vi "Create promotion move.vi"(9 "Destination":T1={"File"=enum."d", "Rank"=enum."4"}, 10 "Source":T1={"File"=enum."d", "Rank"=enum."4"}) -> (3 "Promotion move":refnum<class "Promotion.lvclass">)   [LabVIEW 2016, in "Chesslib.lvlib" / "Promotion.lvclass"]
uses:
  Promotion.lvclass
  C:/Users/GRTaggJ/Documents/Projects/chesslib/Moves/Move/Move.lvclass
  typedef/Square.ctl
  typedef/File.ctl
  typedef/Rank.ctl
  Promotion piece.ctl
  Promotion.lvclass/Promotion.ctl
  Move/Move.lvclass
  Chesslib.lvlib
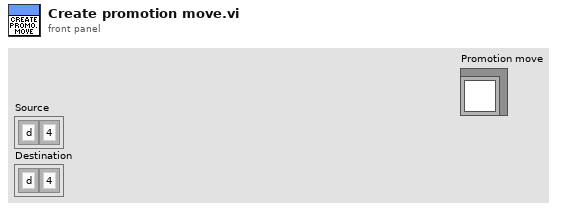
[diagram p1: front panel]
types:
  T1 = typedef "Chesslib.lvlib/Square.ctl" = cluster{"File":T2, "Rank":T3}
  T2 = typedef "Chesslib.lvlib/File.ctl" = enum8{"a", "b", "c", "d", "e", "f", "g", "h"}
  T3 = typedef "Chesslib.lvlib/Rank.ctl" = enum8{"1", "2", "3", "4", "5", "6", "7", "8"}
  T4 = typedef "Chesslib.lvlib/Promotion.lvclass/Promotion piece.ctl" = enum16{"Bishop", "Knight", "Rook", "Queen"}
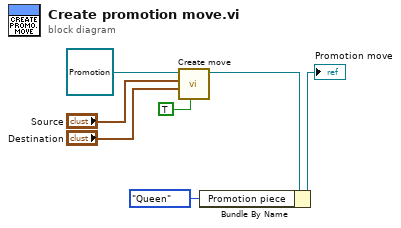
[diagram p0: block diagram]
diagram:
  n1 = call "Create move.vi"("Pawn move (F)"=TRUE, "Destination"="Destination", "Source"="Source", "Move in"=refnum<class "Promotion.lvclass"> refnum ("Promotion in")) -> ("Move out"=w4:refnum<class "Promotion.lvclass">)  [unwired: 7 in]
  n2 = Bundle By Name(cluster=w4, "Promotion piece"=Promotion_piece."Queen") -> (→"Promotion move":refnum<class "Promotion.lvclass">)
